vi "fp display engine.vi"(7 "channel data in":sgl[][][](array[numeric]), 10 "Image Refs In":T1[](array[typedef]), 11 "DisplayRefsIn(generic class)":refnum<vi>[](array[refnum])) -> ()   [LabVIEW 2012]
uses:
  <vilib>/vision/Image Controls.llb/IMAQ Image.ctl
  Custom Controls/MAIN Image panel tab Control type def.ctl
  Custom Controls/Ch selector.ctl
  GFG/GFGfpRefGet.vi
  GFG/GFGbooleanGet.vi
  <vilib>/vision/NI_Vision_Development_Module.lvlib
  GFG/GFG library.lvlib
panel:
  in  "ROI colors":u32[](array[colorbox])=[6618880, 16716362, 16860, 16776793, 16750848, 16448250, 16716530, 9567230, 16764108, 7340212, 32639, 0, 13816530, 8421376, 8421631, 7171459, 6618880, 16716362, 16860, 16776793, 16750848, 16448250, 16716530, 9567230, 16764108, 7340212, 32639, 0, 13816530, 8421376, 8421631, 7171459, 6618880, 16716362, 16860, 16776793, 16750848, 16448250, 16716530, 9567230, 16764108, 7340212, 32639, 0, 13816530, 8421376, 8421631, 7171459, 6618880, 16716362, 16860, 16776793, 16750848, 16448250, 16716530, 9567230, 16764108, 7340212, 32639, 0, 13816530, 8421376, 8421631, 7171459, 6618880, 16716362, 16860, 16776793, 16750848, 16448250, 16716530, 9567230, 16764108, 7340212, 32639, 0, 13816530, 8421376, 8421631, 7171459, 6618880, 16716362, 16860, 16776793, 16750848, 16448250, 16716530, 9567230, 16764108, 7340212, 32639, 0, 13816530, 8421376, 8421631, 7171459, 6618880, 16716362, 16860, 16776793, 16750848, 16448250, 16716530, 9567230, 16764108, 7340212, 32639, 0, 13816530, 8421376, 8421631, 7171459, 6618880, 16716362, 16860, 16776793, 16750848, 16448250, 16716530, 9567230, 16764108, 7340212, 32639, 0, 13816530, 8421376, 8421631, 7171459, 6618880, 16716362, 16860, 16776793, 16750848, 16448250, 16716530, 9567230, 16764108, 7340212, 32639, 0, 13816530, 8421376, 8421631, 7171459, 6618880, 16716362, 16860, 16776793, 16750848, 16448250, 16716530, 9567230, 16764108, 7340212, 32639, 0, 13816530, 8421376, 8421631, 7171459, 6618880, 16716362, 16860, 16776793, 16750848, 16448250, 16716530, 9567230, 16764108, 7340212, 32639, 0, 13816530, 8421376, 8421631, 7171459, 6618880, 16716362, 16860, 16776793, 16750848, 16448250, 16716530, 9567230, 16764108, 7340212, 32639, 0, 13816530, 8421376, 8421631, 7171459, 6618880, 16716362, 16860, 16776793, 16750848, 16448250, 16716530, 9567230, 16764108, 7340212, 32639, 0, 13816530, 8421376, 8421631, 7171459, 6618880, 16716362, 16860, 16776793, 16750848, 16448250, 16716530, 9567230, 16764108, 7340212, 32639, 0, 13816530, 8421376, 8421631, 7171459, 6618880, 16716362, 16860, 16776793, 16750848, 16448250, 16716530, 9567230, 16764108, 7340212, 32639, 0, 13816530, 8421376, 8421631, 7171459, 6618880, 16716362, 16860, 16776793, 16750848, 16448250, 16716530, 9567230, 16764108, 7340212, 32639, 0, 13816530, 8421376, 8421631, 7171459, 6618880, 16716362, 16860, 16776793, 16750848, 16448250, 16716530, 9567230, 16764108, 7340212, 32639, 0, 13816530, 8421376, 8421631, 7171459, 6618880, 16716362, 16860, 16776793, 16750848, 16448250, 16716530, 9567230, 16764108, 7340212, 32639, 0, 13816530, 8421376, 8421631, 7171459, 6618880, 16716362, 16860, 16776793, 16750848, 16448250, 16716530, 9567230, 16764108, 7340212, 32639, 0, 13816530, 8421376, 8421631, 7171459, 6618880, 16716362, 16860, 16776793, 16750848, 16448250, 16716530, 9567230, 16764108, 7340212, 32639, 0, 13816530, 8421376, 8421631, 7171459, 6618880, 16716362, 16860, 16776793, 16750848, 16448250, 16716530, 9567230, 16764108, 7340212, 32639, 0, 13816530, 8421376, 8421631, 7171459, 6618880, 16716362, 16860, 16776793, 16750848, 16448250, 16716530, 9567230, 16764108, 7340212, 32639, 0, 13816530, 8421376, 8421631, 7171459, 6618880, 16716362, 16860, 16776793, 16750848, 16448250, 16716530, 9567230, 16764108, 7340212, 32639, 0, 13816530, 8421376, 8421631, 7171459, 6618880, 16716362, 16860, 16776793, 16750848, 16448250, 16716530, 9567230, 16764108, 7340212, 32639, 0, 13816530, 8421376, 8421631, 7171459, 6618880, 16716362, 16860, 16776793, 16750848, 16448250, 16716530, 9567230, 16764108, 7340212, 32639, 0, 13816530, 8421376, 8421631, 7171459]
  out "error out":errorcluster
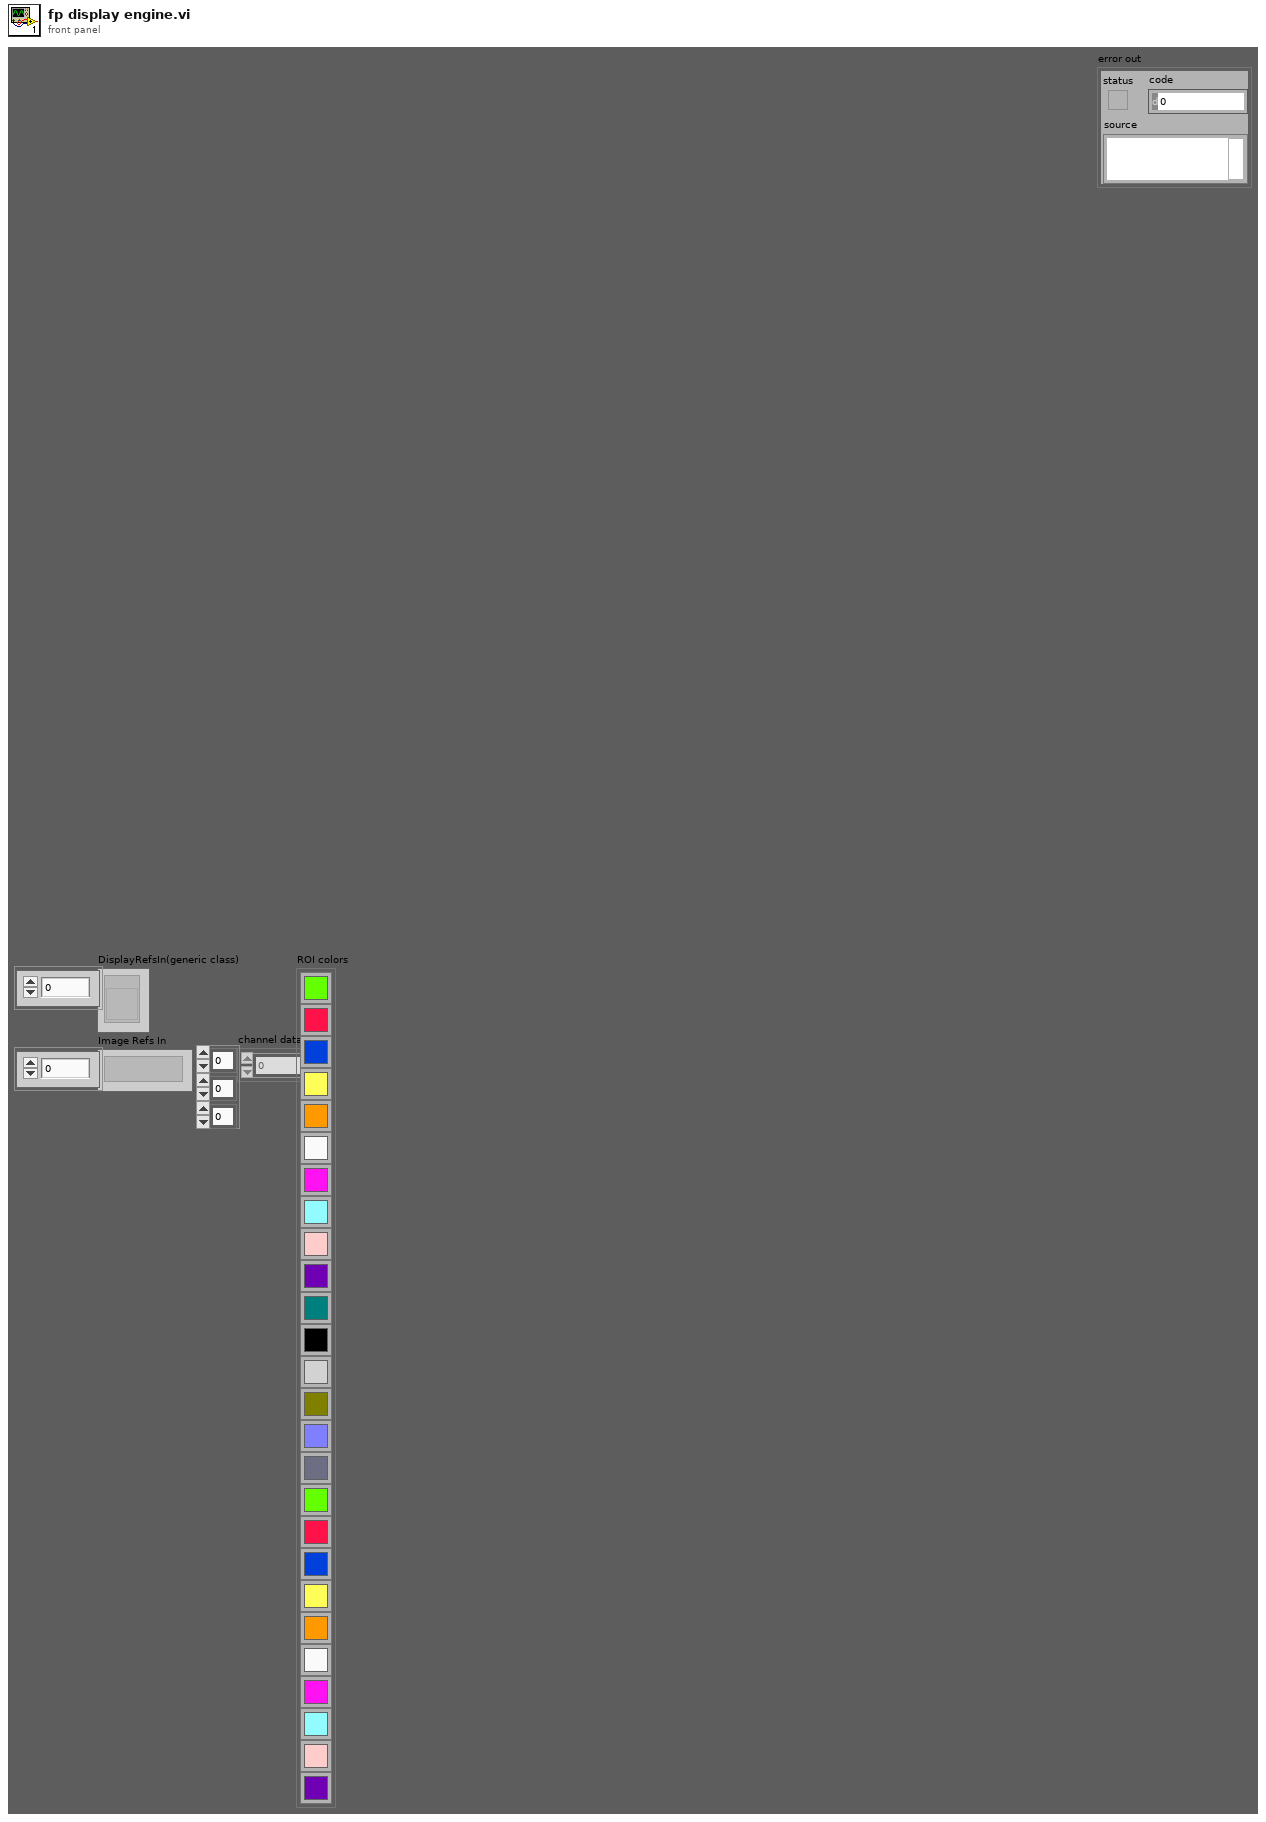
[diagram p1: front panel]
types:
  T1 = typedef "IMAQ Image.ctl" = refnum<image>
  T2 = typedef "MAIN Image panel tab Control type def.ctl" = enum32{"Channel 1", "Channel 2", "Channel 3", "Channel 4", "all channels", "RGB overlay", "ROI", "arbitrary line scan"}
  T3 = enum32{"Channel 1", "Channel 2", "Channel 3", "Channel 4", "Channel 5", "all channels", "RGB overlay", "ROI", "arbitrary line scan"}
  T4 = typedef "Ch selector.ctl" = enum16{"none", "Ch 1", "Ch 2", "Ch 3", "Ch 4", "Ch 5"}
  T5 = typedef "Image Type" = u32
  T6 = cluster{"Global Rectangle":i32[], "Contours":cluster{"Contour Type":u32, "ROI Type":u32, "Points":i32[]}[]}
  T7 = typedef "ROI Descriptor" = cluster{"Global Rectangle":i32[], "Contours":cluster{"ID":enum32{"External", "Internal"}, "Type":u32, "Coordinates":i32[]}[]}
  T8 = cluster{"WaveformChartRef":refnum<vi>, "DigitalRef":refnum<vi>, "ArrayRef":refnum<vi>, "TabControlRef":refnum<vi>, "EnumRef":refnum<vi>, "RingRef":refnum<vi>, "BooleanRef":refnum<vi>, "KnobRef":refnum<vi>, "SlideRef":refnum<vi>, "PathRef":refnum<vi>, "StringRef":refnum<vi>, "ComboBox":refnum<vi>, "WaveformGraphRef":refnum<vi>}
  T9 = cluster{"Mean Value":sgl, "Standard Variation":sgl, "Minimal Value":sgl, "Maximal Value":sgl, "Area (calibrated)":sgl, "Area (pixels)":i32, "%":sgl}[]
  T10 = cluster{"Mean Value":sgl, "Standard Variation":sgl, "Minimal Value":sgl, "Maximal Value":sgl, "Area (calibrated)":sgl, "Area (pixels)":i32, "%":sgl}
  T11 = cluster{"Contour Type":u32, "ROI Type":u32, "Points":i32[]}[]
  T12 = cluster{"Starting Value":sgl, "Incremental Value":sgl, "Histogram":u32[]}
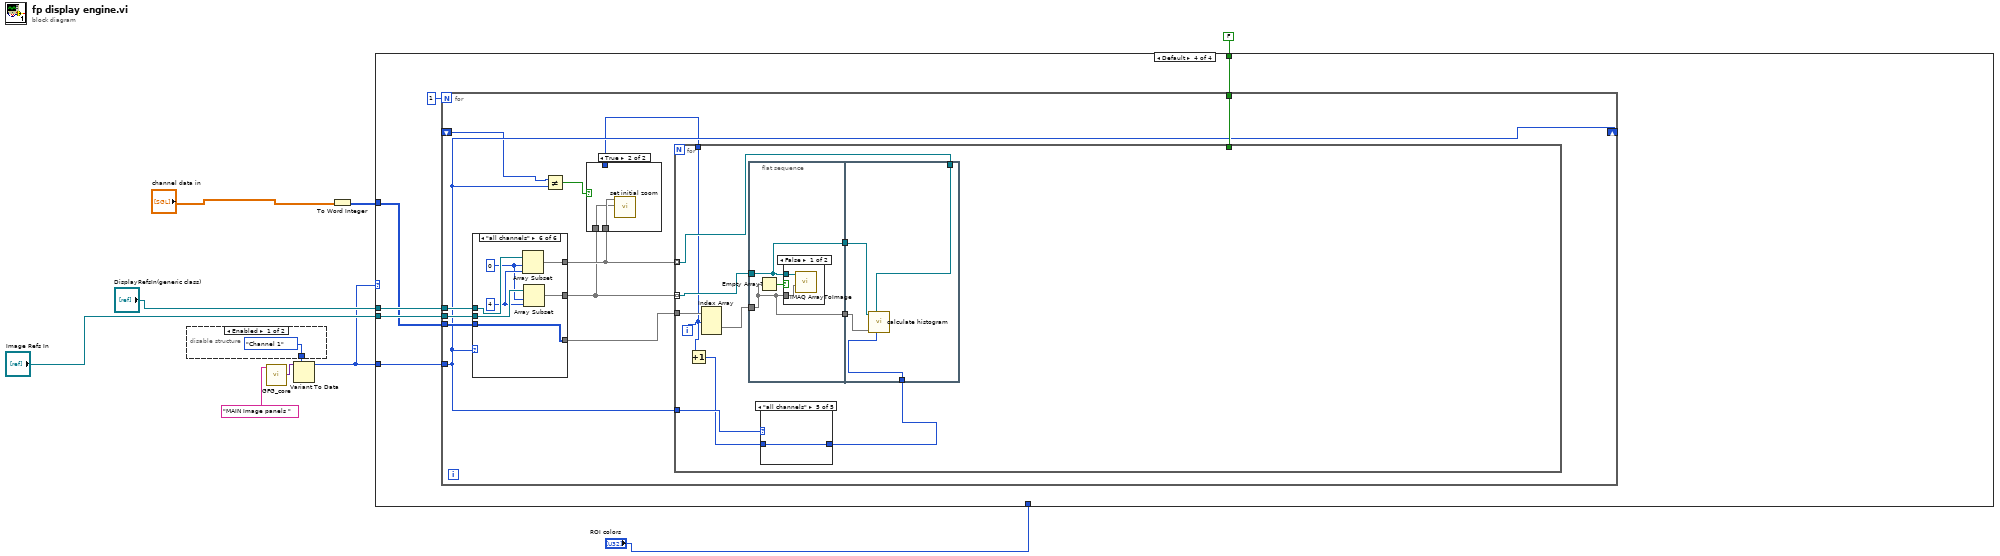
[diagram p0: block diagram]
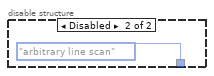
[diagram p2: hidden frame]
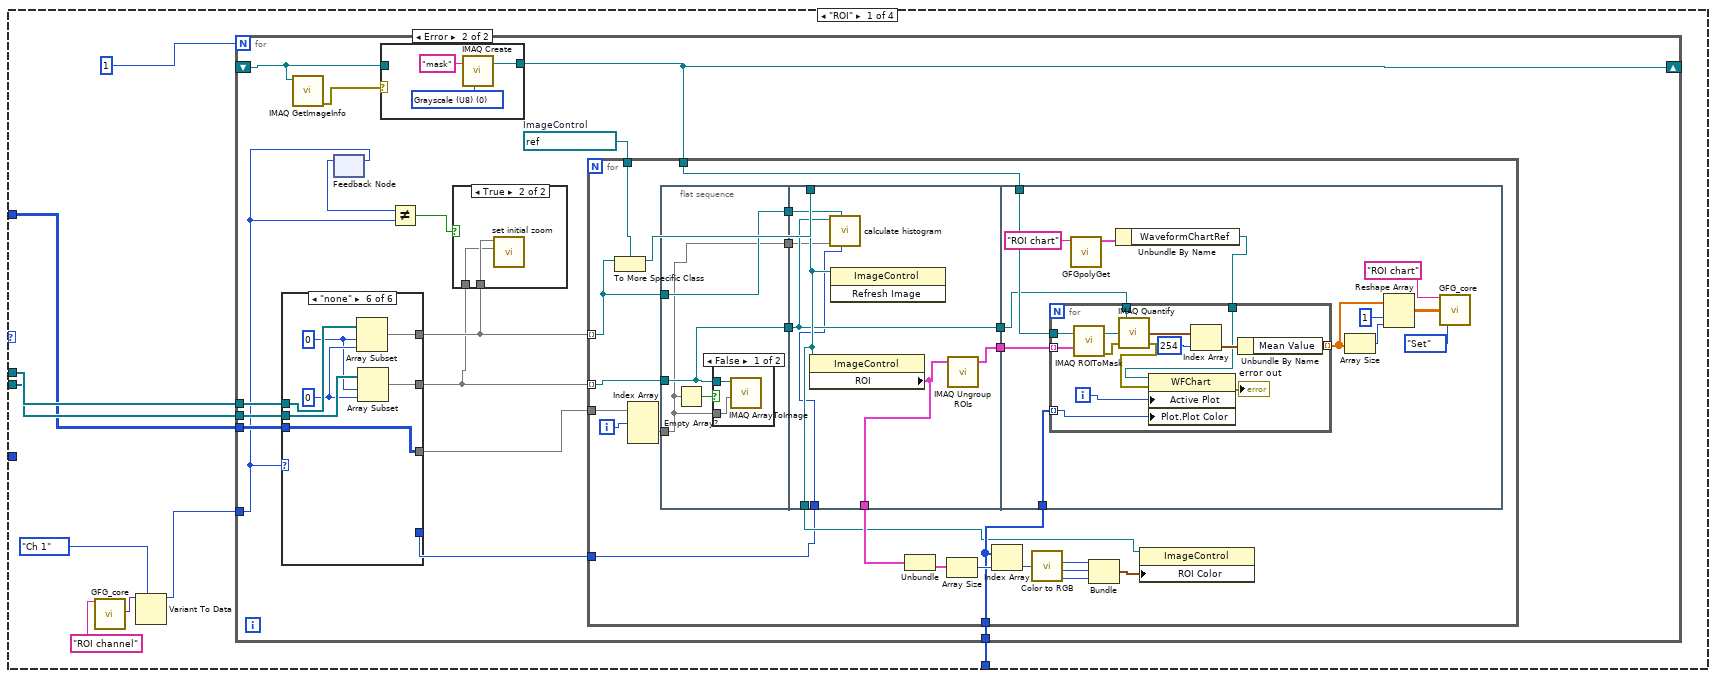
[diagram p3: hidden frame]
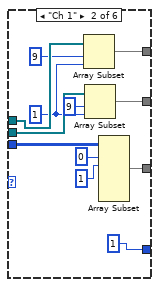
[diagram p7: hidden frame]
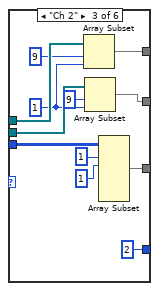
[diagram p8: hidden frame]
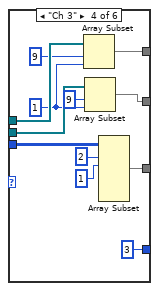
[diagram p9: hidden frame]
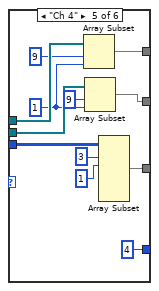
[diagram p10: hidden frame]
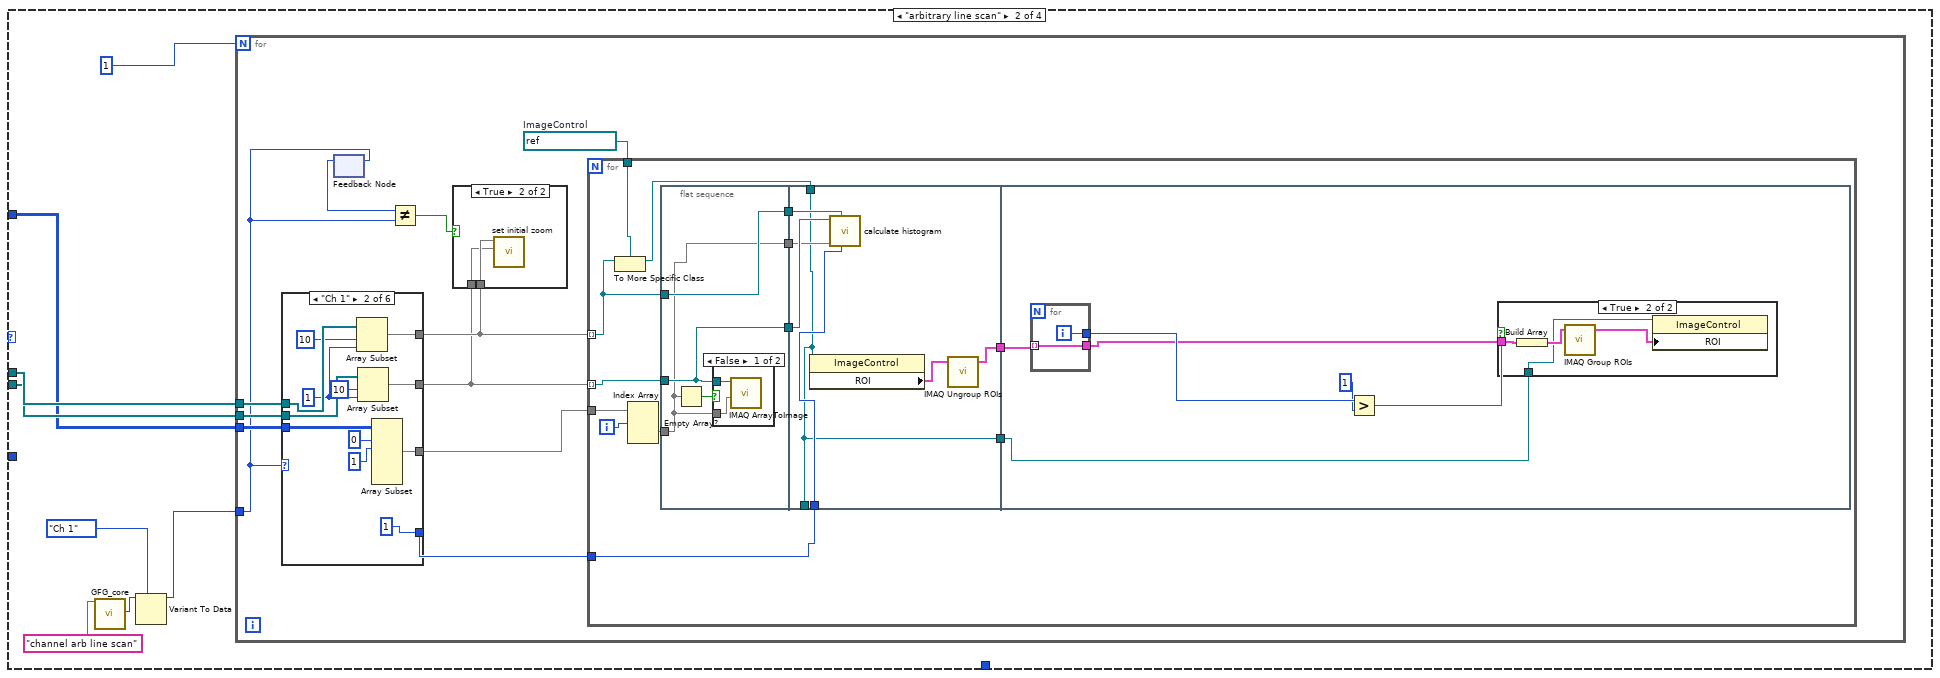
[diagram p12: hidden frame]
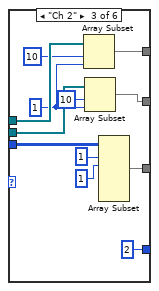
[diagram p15: hidden frame]
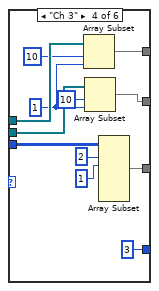
[diagram p16: hidden frame]
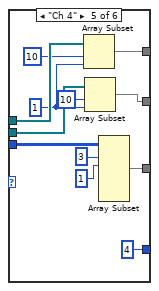
[diagram p17: hidden frame]
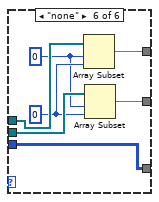
[diagram p18: hidden frame]
diagram:
  n1 = disable-structure shown="Enabled" {
    disable-tunnel: [MAIN_Image_panel_tab_Control_type_def."Channel 1" ("MAIN Image panels") T3."arbitrary line scan" ("MAIN Image panels")] -> w8
    frame Enabled {
    }
    frame Disabled {
    }
  }
  n2 = call "GFG_core.vi"("Variable Name in"="MAIN Image panels ") -> ("Variant Out"=w10:variant)  [unwired: 12 in, 6 out]
  n3 = Variant To Data(type=w8, Variant=w10) -> (data=w4:T2)  [unwired: 1 in, 1 out]
  n4 = To Word Integer(number="channel data in") -> (16bit integer=w3:i16[][][])
  n5 = case shown="Default" w4 {
    tunnel: w4 -> [_ _ _ w356]
    tunnel: "DisplayRefsIn(generic class)" -> [w20 w168 w290 w359]
    tunnel: "Image Refs In" -> [w19 w167 w281 w358]
    tunnel: w3 -> [w18 w166 w289 w357]
    tunnel: FALSE -> [_ _ w288 w354]
    tunnel: "ROI colors" -> [w14 _ _ _]
    frame "ROI" {
      n6 = call "GFG_core.vi"("Variable Name in"="ROI channel") -> ("Variant Out"=w16:variant)  [unwired: 12 in, 6 out]
      n7 = Variant To Data(type=Ch_selector."Ch 1" ("ROI channel"), Variant=w16) -> (data=w15:T4)  [unwired: 1 in, 1 out]
      n8 = for {
        N: 1 -> [_]
        tunnel: w20 -> [w35]
        tunnel: w19 -> [w34]
        tunnel: w18 -> [w33]
        tunnel: w15 -> [w30]
        shift-right: [w27] -> _
        shift-left: _ -> [w26]
        tunnel: w14 -> [w24]
        w32 = refnum<vi> refnum  # ImageControl
        n9 = case shown="\"none\"" w30 {
          tunnel: w35 -> [_ w53 w65 w77 w89 w96]
          tunnel: w34 -> [_ w54 w66 w78 w90 w97]
          tunnel: [_ w50 w62 w74 w86 w93] -> w22
          tunnel: [_ w49 w61 w73 w85 w92] -> w29
          tunnel: w33 -> [_ w48 w58 w70 w82 w91]
          tunnel: [_ w45 w57 w69 w81 w91] -> w36
          tunnel: [_ 1 ("length") 2 ("length") 3 ("length") 4 ("length") _] -> w23
          frame Default {
          }
          frame "Ch 1" {
            w52 = 1 ("length")
            n10 = Array Subset(array=w53, index=9, length=w52) -> (w49:refnum<vi>[])
            n11 = Array Subset(array=w54, index=9, length=w52) -> (w50:T1[])
            n12 = Array Subset(array=w48, index (dim 0)=0 ("index"), length (dim 0)=1 ("length")) -> (w45:i16[][][])  [unwired: 4 in]
          }
          frame "Ch 2" {
            w64 = 1 ("length")
            n13 = Array Subset(array=w65, index=9, length=w64) -> (w61:refnum<vi>[])
            n14 = Array Subset(array=w66, index=9, length=w64) -> (w62:T1[])
            n15 = Array Subset(array=w58, index (dim 0)=1 ("index"), length (dim 0)=1 ("length")) -> (w57:i16[][][])  [unwired: 4 in]
          }
          frame "Ch 3" {
            w75 = 1 ("index")
            n16 = Array Subset(array=w77, index=9, length=w75) -> (w73:refnum<vi>[])
            n17 = Array Subset(array=w78, index=9, length=w75) -> (w74:T1[])
            n18 = Array Subset(array=w70, index (dim 0)=2 ("index"), length (dim 0)=1 ("length")) -> (w69:i16[][][])  [unwired: 4 in]
          }
          frame "Ch 4" {
            w88 = 1 ("index")
            n19 = Array Subset(array=w89, index=9, length=w88) -> (w85:refnum<vi>[])
            n20 = Array Subset(array=w90, index=9, length=w88) -> (w86:T1[])
            n21 = Array Subset(array=w82, index (dim 0)=3 ("index"), length (dim 0)=1 ("length")) -> (w81:i16[][][])  [unwired: 4 in]
          }
          frame "none" {
            w94 = 0 ("index")
            w95 = 0 ("length")
            n22 = Array Subset(array=w96, index=w94, length=w95) -> (w92:refnum<vi>[])
            n23 = Array Subset(array=w97, index=w94, length=w95) -> (w93:T1[])
          }
        }
        n24 = call "IMAQ GetImageInfo"("Image"=w26) -> ("error out"=w25:errorcluster)  [unwired: 3 in, 7 out]
        n25 = feedback-in #1(w30) -> ()
        n26 = feedback #1() -> (w31:T4)  [unwired: 1 in]
        n27 = case shown="Error" w25 {
          tunnel: [w37 w38] -> w27
          tunnel: w26 -> [w37 _]
          frame No Error {
          }
          frame Error {
            w39 = T5 0 items=["Grayscale (U8)", "Grayscale (I16)", "Grayscale (SGL)", "Complex (CSG)", "RGB (U32)", "HSL (U32)", "RGB (U64)"] ("Image Type")
            n28 = call "IMAQ Create"("Image Name"="mask", "Image Type"=w39) -> ("New Image"=w38:T1)  [unwired: 3 in, 1 out]
          }
        }
        n29 = Not Equal?(x=w31, y=w30) -> (x != y?=w28:bool)
        n30 = case shown="True" w28 {
          tunnel: w29 -> [_ w42]
          tunnel: w22 -> [_ w41]
          frame False {
          }
          frame True {
            n31 = call "set initial zoom.vi"("Image Refs In"=w41, "DisplayRefsIn(generic class)"=w42) -> ()  [unwired: 10 in]
          }
        }
        n32 = for {
          tunnel: w29 -> [w100] mode=indexing
          tunnel: w22 -> [w119] mode=indexing
          tunnel: w36 -> [w121]
          tunnel: w32 -> [w118]
          tunnel: w27 -> [w103]
          tunnel: w24 -> [w106]
          tunnel: w23 -> [w98]
          i -> [w116]
          n33 = To More Specific Class(target class=w118, reference=w100) -> (specific class reference=w117:refnum<vi>)  [unwired: 1 in, 1 out]
          n34 = Index Array(array=w121, index (dim 0)=w116) -> (element=w120:i16[][])  [unwired: 2 in]
          n35 = flat-sequence {
            tunnel: w120 -> [w122]
            tunnel: w119 -> [w124]
            tunnel: [w124] -> w104
            tunnel: [w123] -> w101
            tunnel: w100 -> [w123]
            tunnel: [w122] -> w99
            tunnel: w117 -> [w132]
            tunnel: [w134] -> w109
            tunnel: [w133] -> w107
            tunnel: [w130] -> w105
            tunnel: w104 -> [w130]
            tunnel: [w132] -> w102
            tunnel: w101 -> [w131]
            tunnel: w99 -> [w129]
            tunnel: w98 -> [w128]
            tunnel: w107 -> [w144]
            tunnel: w106 -> [w143]
            tunnel: w105 -> [w135]
            tunnel: w103 -> [w136]
            frame #0 {
              n36 = Empty Array?(array=w122) -> (empty?=w125:bool)
              n37 = case shown="False" w125 {
                tunnel: w124 -> [w127 _]
                tunnel: w122 -> [w126 _]
                frame False {
                  n38 = call "IMAQ ArrayToImage"("Image Pixels (I16)"=w126, "Image"=w127) -> ()  [unwired: 8 in, 2 out]
                }
                frame True {
                }
              }
            }
            frame #1 {
              n39 = property class="ImageControl"(reference=w132) -> ("ROI"=w134:T6)  [unwired: 1 in, 2 out]
              n40 = call "calculate histogram.vi"("channel no."=w128, "Image Ctrl Ref (as generic class)"=w131, "Image Array"=w129, "Image"=w130) -> ()  [unwired: 8 in]
              n41 = invoke class="ImageControl" method="Refresh Image"(reference=w132) -> ()  [unwired: 2 in, 3 out]
              n42 = call "IMAQ Ungroup ROIs"("ROI Descriptor"=w134) -> ("ROI Descriptors out"=w133:T7[])  [unwired: 3 in, 1 out]
            }
            frame #2 {
              n43 = call-poly "GFGpolyGet.vi"("Variable Name in"="ROI chart") -> ("output cluster"=w138:T8)  [unwired: 9 in, 1 out]
              n44 = Unbundle By Name(w138) -> ("WaveformChartRef"=w137:refnum<vi>)
              n45 = for {
                tunnel: w135 -> [w161]
                tunnel: w144 -> [w155] mode=indexing
                tunnel: [w157] -> w147 mode=indexing
                tunnel: w136 -> [w154]
                tunnel: w143 -> [w151] mode=indexing
                tunnel: w137 -> [w150]
                i -> [w152]
                n46 = call "IMAQ ROIToMask"("ROI Descriptor"=w155, "Image"=w154) -> ("error out"=w149:errorcluster, "Image Out"=w156:T1)  [unwired: 4 in, 1 out]
                n47 = call "IMAQ Quantify"("error in (no error)"=w149, "Image Mask"=w156, "Image"=w161) -> ("error out"=w148:errorcluster, "Region Reports"=w160:T9)  [unwired: 1 out]
                n48 = property on="Property Node" class="WFChart"(reference=w150, error in=w148, "Active Plot"=w152, "Plot.Plot Color"=w151) -> (error out=→"error out":errorcluster)  [unwired: 1 out]
                n49 = Index Array(array=w160, index=254) -> (element=w158:T10)
                n50 = Unbundle By Name(w158) -> ("Mean Value"=w157:sgl)
              }
              n51 = Array Size(array=w147) -> (size(s)=w146:i32)
              n52 = Reshape Array(w147, 1 ("dimension size"), w146) -> (w141:sgl[][])
              n53 = call "GFG_core.vi"("Variable Name in"="ROI chart", "Variant in"=w141, "Action"=enum16{"Init", "Set", "Get"}."Set") -> ()  [unwired: 10 in, 7 out]
            }
          }
          n54 = Unbundle(w109) -> ("Contours"=w114:T11)  [unwired: 1 out]
          n55 = Array Size(array=w114) -> (size(s)=w115:i32)
          n56 = Index Array(array=w106, index=w115) -> (element=w110:u32)
          n57 = call <vilib>:"Color to RGB.vi"("Color"=w110) -> ("R"=w111:u8, "G"=w112:u8, "B"=w113:u8)  [unwired: 1 out]
          n58 = Bundle("R"=w111, "G"=w112, "B"=w113) -> (w108:cluster{"R":u8, "G":u8, "B":u8})  [unwired: 1 in]
          n59 = property class="ImageControl"(reference=w102, "ROI Color"=w108) -> ()  [unwired: 1 in, 2 out]
        }
      }
    }
    frame "arbitrary line scan" {
      n60 = call "GFG_core.vi"("Variable Name in"="channel arb line scan") -> ("Variant Out"=w164:variant)  [unwired: 12 in, 6 out]
      n61 = Variant To Data(type=Ch_selector."Ch 1" ("ROI channel"), Variant=w164) -> (data=w163:T4)  [unwired: 1 in, 1 out]
      n62 = for {
        N: 1 -> [_]
        tunnel: w168 -> [w179]
        tunnel: w167 -> [w178]
        tunnel: w166 -> [w177]
        tunnel: w163 -> [w174]
        w176 = refnum<vi> refnum  # ImageControl
        n63 = case shown="\"Ch 1\"" w174 {
          tunnel: w179 -> [_ w193 w205 w217 w229 w236]
          tunnel: w178 -> [_ w194 w206 w218 w230 w237]
          tunnel: [_ w190 w202 w214 w226 w233] -> w170
          tunnel: [_ w189 w201 w213 w225 w232] -> w173
          tunnel: w177 -> [_ w188 w198 w210 w222 w231]
          tunnel: [_ w185 w197 w209 w221 w231] -> w180
          tunnel: [_ 1 ("length") 2 ("length") 3 ("length") 4 ("length") _] -> w171
          frame Default {
          }
          frame "Ch 1" {
            w192 = 1 ("length")
            n64 = Array Subset(array=w193, index=10, length=w192) -> (w189:refnum<vi>[])
            n65 = Array Subset(array=w194, index=10, length=w192) -> (w190:T1[])
            n66 = Array Subset(array=w188, index (dim 0)=0 ("index"), length (dim 0)=1 ("length")) -> (w185:i16[][][])  [unwired: 4 in]
          }
          frame "Ch 2" {
            w204 = 1 ("length")
            n67 = Array Subset(array=w205, index=10, length=w204) -> (w201:refnum<vi>[])
            n68 = Array Subset(array=w206, index=10, length=w204) -> (w202:T1[])
            n69 = Array Subset(array=w198, index (dim 0)=1 ("index"), length (dim 0)=1 ("length")) -> (w197:i16[][][])  [unwired: 4 in]
          }
          frame "Ch 3" {
            w215 = 1 ("index")
            n70 = Array Subset(array=w217, index=10, length=w215) -> (w213:refnum<vi>[])
            n71 = Array Subset(array=w218, index=10, length=w215) -> (w214:T1[])
            n72 = Array Subset(array=w210, index (dim 0)=2 ("index"), length (dim 0)=1 ("length")) -> (w209:i16[][][])  [unwired: 4 in]
          }
          frame "Ch 4" {
            w228 = 1 ("index")
            n73 = Array Subset(array=w229, index=10, length=w228) -> (w225:refnum<vi>[])
            n74 = Array Subset(array=w230, index=10, length=w228) -> (w226:T1[])
            n75 = Array Subset(array=w222, index (dim 0)=3 ("index"), length (dim 0)=1 ("length")) -> (w221:i16[][][])  [unwired: 4 in]
          }
          frame "none" {
            w234 = 0 ("index")
            w235 = 0 ("length")
            n76 = Array Subset(array=w236, index=w234, length=w235) -> (w232:refnum<vi>[])
            n77 = Array Subset(array=w237, index=w234, length=w235) -> (w233:T1[])
          }
        }
        n78 = feedback-in #2(w174) -> ()
        n79 = feedback #2() -> (w175:T4)  [unwired: 1 in]
        n80 = Not Equal?(x=w175, y=w174) -> (x != y?=w172:bool)
        n81 = case shown="True" w172 {
          tunnel: w173 -> [_ w182]
          tunnel: w170 -> [_ w181]
          frame False {
          }
          frame True {
            n82 = call "set initial zoom.vi"("Image Refs In"=w181, "DisplayRefsIn(generic class)"=w182) -> ()  [unwired: 10 in]
          }
        }
        n83 = for {
          tunnel: w173 -> [w241] mode=indexing
          tunnel: w170 -> [w248] mode=indexing
          tunnel: w180 -> [w250]
          tunnel: w176 -> [w247]
          tunnel: w171 -> [w239]
          i -> [w245]
          n84 = To More Specific Class(target class=w247, reference=w241) -> (specific class reference=w246:refnum<vi>)  [unwired: 1 in, 1 out]
          n85 = Index Array(array=w250, index (dim 0)=w245) -> (element=w249:i16[][])  [unwired: 2 in]
          n86 = flat-sequence {
            tunnel: w249 -> [w251]
            tunnel: w248 -> [w253]
            tunnel: [w253] -> w243
            tunnel: [w252] -> w242
            tunnel: w241 -> [w252]
            tunnel: [w251] -> w240
            tunnel: w246 -> [w258]
            tunnel: [w263] -> w244
            tunnel: w243 -> [w261]
            tunnel: [w258] -> _
            tunnel: w242 -> [w262]
            tunnel: w240 -> [w260]
            tunnel: w239 -> [w259]
            tunnel: [w258] -> w238
            tunnel: w244 -> [w269]
            tunnel: w238 -> [w268]
            frame #0 {
              n87 = Empty Array?(array=w251) -> (empty?=w254:bool)
              n88 = case shown="False" w254 {
                tunnel: w253 -> [w256 _]
                tunnel: w251 -> [w255 _]
                frame False {
                  n89 = call "IMAQ ArrayToImage"("Image Pixels (I16)"=w255, "Image"=w256) -> ()  [unwired: 8 in, 2 out]
                }
                frame True {
                }
              }
            }
            frame #1 {
              n90 = property class="ImageControl"(reference=w258) -> ("ROI"=w257:T6)  [unwired: 1 in, 2 out]
              n91 = call "calculate histogram.vi"("channel no."=w259, "Image Ctrl Ref (as generic class)"=w262, "Image Array"=w260, "Image"=w261) -> ()  [unwired: 8 in]
              n92 = call "IMAQ Ungroup ROIs"("ROI Descriptor"=w257) -> ("ROI Descriptors out"=w263:T7[])  [unwired: 3 in, 1 out]
            }
            frame #2 {
              n93 = for {
                tunnel: w269 -> [w275] mode=indexing
                tunnel: [w275] -> w264
                tunnel: [w274] -> w267
                i -> [w274]
              }
              n94 = Greater?(x=w267, y=1) -> (0:w265:bool)
              n95 = case shown="True" w265 {
                tunnel: w264 -> [_ w273]
                tunnel: w268 -> [_ w270]
                frame False {
                }
                frame True {
                  n96 = Build Array(w273) -> (w272:T7[])
                  n97 = call "IMAQ Group ROIs"("ROI Descriptors"=w272) -> ("ROI Descriptor out"=w271:T7)  [unwired: 3 in, 1 out]
                  n98 = property class="ImageControl"(reference=w270, "ROI"=w271) -> ()  [unwired: 1 in, 2 out]
                }
              }
            }
          }
        }
      }
    }
    frame "RGB overlay" {
      w276 = refnum<vi> refnum  # ImageControl
      n99 = Array Subset(array=w281, index=8, length=1) -> (w280:T1[])
      n100 = Array Subset(array=w290, index=8, length=1) -> (w277:refnum<vi>[])
      n101 = Array Subset(array=w281, index=0, length=4) -> (w278:T1[])
      n102 = call "set initial zoom.vi"("Image Refs In"=w278, "DisplayRefsIn(generic class)"=w277) -> ()  [unwired: 10 in]
      n103 = for {
        tunnel: w278 -> [w310] mode=indexing
        tunnel: w289 -> [w312]
        tunnel: w288 -> [w303]
        tunnel: [w299] -> w279 mode=indexing
        i -> [w307]
        n104 = Increment(x=w307) -> (x+1=w305:i32)
        n105 = Index Array(array=w312, index (dim 0)=w307) -> (element=w311:i16[][])  [unwired: 2 in]
        n106 = flat-sequence {
          tunnel: w311 -> [w313]
          tunnel: w310 -> [w314]
          tunnel: [w314] -> w308
          tunnel: [w313] -> w306
          tunnel: [w323] -> w309
          tunnel: w308 -> [w323]
          tunnel: w306 -> [w318]
          tunnel: [w321] -> w304
          tunnel: [w318] -> w302
          tunnel: w309 -> [w342]
          tunnel: w305 -> [w341]
          tunnel: w304 -> [w329]
          tunnel: w303 -> [w324]
          tunnel: [w326] -> w300
          tunnel: [w325] -> w301
          frame #0 {
            n107 = Empty Array?(array=w313) -> (empty?=w315:bool)
            n108 = case shown="False" w315 {
              tunnel: w314 -> [w317 _]
              tunnel: w313 -> [w316 _]
              frame False {
                n109 = call "IMAQ ArrayToImage"("Image Pixels (I16)"=w316, "Image"=w317) -> ()  [unwired: 8 in, 2 out]
              }
              frame True {
              }
            }
          }
          frame #1 {
            n110 = Array Max & Min(array=w318) -> (max value=w322:i16, min value=w320:i16)  [unwired: 2 out]
            n111 = Decrement(x=w322) -> (x-1=w319:i16)
            n112 = Bundle(w320, w319) -> (w321:cluster{i16, i16})  [unwired: 1 in]
          }
          frame #2 {
            n113 = Number To Decimal String(number=w341) -> (decimal integer string=w336:string)  [unwired: 1 in]
            n114 = Concatenate Strings("Histogram " ("string"), w336) -> (w344:string)
            n115 = Concatenate Strings("auto scale\n      CH " ("Variable Name in"), w336) -> (w339:string)
            n116 = Concatenate Strings("Min Max Channel " ("Variable Name in"), w336) -> (w327:string)
            n117 = call "IMAQ Histograph"("Image"=w342) -> ("Histogram Graph"=w347:T12)  [unwired: 7 in, 3 out]
            n118 = call-poly "GFGpolyGet.vi"("Variable Name in"=w327) -> ("output cluster"=w338:T8)  [unwired: 9 in, 1 out]
            n119 = call-poly "GFGpolyGet.vi"("Variable Name in"=w339) -> ("Boolean"=w332:bool)  [unwired: 10 in]
            n120 = call-poly "GFGpolyGet.vi"("Variable Name in"=w344) -> ("output cluster"=w345:T8)  [unwired: 9 in, 1 out]
            n121 = Unbundle By Name(w345) -> ("WaveformGraphRef"=w346:refnum<vi>)
            n122 = Unbundle By Name(w338) -> ("SlideRef"=w335:refnum<vi>)
            n123 = property class="WFGraph"(reference=w346, "Value"=w347) -> ()  [unwired: 1 in, 2 out]
            n124 = property class="Slide"(reference=w335) -> (reference out=w330:refnum<vi>, "Value"=w334:variant)  [unwired: 1 in, 1 out]
            n125 = Variant To Data(type=cluster{i32, i32} {0, 2048} ("channel1"), Variant=w334) -> (data=w331:cluster{i32, i32})  [unwired: 1 in, 1 out]
            n126 = Select(t=w329, s=w332, f=w331) -> (s? t:f=w328:cluster{i32, i32})
            n127 = case shown="False" w324 {
              tunnel: w328 -> [w350 w353]
              tunnel: [w349 w351] -> w326
              tunnel: [w348 w352] -> w325
              frame True {
                n128 = Unbundle(w350) -> (w349:i32, w348:i32)
              }
              frame False {
                n129 = Unbundle(w353) -> (w352:i32, w351:i32)
              }
            }
            n130 = property class="Slide"(reference=w330, "Value"=w328) -> ()  [unwired: 1 in, 2 out]
          }
        }
        n131 = Bundle(w302, w301, w300) -> (w299:cluster{i16[][], i32, i32})  [unwired: 1 in]
      }
      n132 = for {
        tunnel: w280 -> [w295] mode=indexing
        tunnel: w279 -> [w294]
        tunnel: w277 -> [w293] mode=indexing
        tunnel: w276 -> [w292]
        n133 = flat-sequence {
          tunnel: w295 -> [w297]
          tunnel: w294 -> [w296]
          tunnel: w291 -> [w298]
          frame #0 {
            n134 = call "overlay3channels.vi"("RGB Overlay"=w297, "Array"=w296) -> ()  [unwired: 10 in]
          }
          frame #1 {
            n135 = invoke class="ImageControl" method="Refresh Image"(reference=w298) -> ()  [unwired: 2 in, 3 out]
          }
        }
        n136 = To More Specific Class(target class=w292, reference=w293) -> (specific class reference=w291:refnum<vi>)  [unwired: 1 in, 1 out]
      }
    }
    frame Default {
      n137 = for {
        N: 1 -> [_]
        tunnel: w359 -> [w369]
        tunnel: w358 -> [w368]
        tunnel: w357 -> [w367]
        tunnel: w356 -> [w362]
        tunnel: w354 -> [w364]
        shift-right: [w362] -> _
        shift-left: _ -> [w361]
        n138 = case shown="\"all channels\"" w362 {
          tunnel: w369 -> [_ w381 w391 w401 w411 w418]
          tunnel: w368 -> [_ w382 w392 w402 w412 w419]
          tunnel: [_ w378 w388 w398 w408 w415] -> w363
          tunnel: [_ w377 w387 w397 w407 w414] -> w366
          tunnel: w367 -> [_ w376 w384 w394 w404 w413]
          tunnel: [_ w373 w383 w393 w403 w413] -> w370
          frame Default {
          }
          frame "Channel 1" {
            w379 = 4 ("index")
            w380 = 1 ("length")
            n139 = Array Subset(array=w381, index=w379, length=w380) -> (w377:refnum<vi>[])
            n140 = Array Subset(array=w382, index=w379, length=w380) -> (w378:T1[])
            n141 = Array Subset(array=w376, index (dim 0)=0 ("index"), length (dim 0)=1 ("length")) -> (w373:i16[][][])  [unwired: 4 in]
          }
          frame "Channel 2" {
            w389 = 5 ("index")
            w390 = 1 ("length")
            n142 = Array Subset(array=w391, index=w389, length=w390) -> (w387:refnum<vi>[])
            n143 = Array Subset(array=w392, index=w389, length=w390) -> (w388:T1[])
            n144 = Array Subset(array=w384, index (dim 0)=1 ("index"), length (dim 0)=1 ("length")) -> (w383:i16[][][])  [unwired: 4 in]
          }
          frame "Channel 3" {
            w399 = 1 ("index")
            w400 = 6 ("index")
            n145 = Array Subset(array=w401, index=w400, length=w399) -> (w397:refnum<vi>[])
            n146 = Array Subset(array=w402, index=w400, length=w399) -> (w398:T1[])
            n147 = Array Subset(array=w394, index (dim 0)=2 ("index"), length (dim 0)=1 ("length")) -> (w393:i16[][][])  [unwired: 4 in]
          }
          frame "Channel 4" {
            w409 = 7 ("index")
            w410 = 1 ("index")
            n148 = Array Subset(array=w411, index=w409, length=w410) -> (w407:refnum<vi>[])
            n149 = Array Subset(array=w412, index=w409, length=w410) -> (w408:T1[])
            n150 = Array Subset(array=w404, index (dim 0)=3 ("index"), length (dim 0)=1 ("length")) -> (w403:i16[][][])  [unwired: 4 in]
          }
          frame "all channels" {
            w416 = 0 ("index")
            w417 = 4 ("length")
            n151 = Array Subset(array=w418, index=w416, length=w417) -> (w414:refnum<vi>[])
            n152 = Array Subset(array=w419, index=w416, length=w417) -> (w415:T1[])
          }
        }
        n153 = Not Equal?(x=w361, y=w362) -> (x != y?=w365:bool)
        n154 = for {
          tunnel: w366 -> [w421] mode=indexing
          tunnel: w363 -> [w424] mode=indexing
          tunnel: w370 -> [w429]
          tunnel: w362 -> [w428]
          tunnel: w364 -> [_]
          tunnel: [w420] -> w360
          i -> [w420]
          n155 = Increment(x=w420) -> (x+1=w427:i32)
          n156 = Index Array(array=w429, index (dim 0)=w420) -> (element=w423:i16[][])  [unwired: 2 in]
          n157 = flat-sequence {
            tunnel: w423 -> [w430]
            tunnel: w424 -> [w431]
            tunnel: [w431] -> w426
            tunnel: [w430] -> w425
            tunnel: w426 -> [w436]
            tunnel: w425 -> [w438]
            tunnel: w422 -> [w437]
            tunnel: w421 -> [w435]
            frame #0 {
              n158 = Empty Array?(array=w430) -> (empty?=w432:bool)
              n159 = case shown="False" w432 {
                tunnel: w431 -> [w434 _]
                tunnel: w430 -> [w433 _]
                frame False {
                  n160 = call "IMAQ ArrayToImage"("Image Pixels (I16)"=w433, "Image"=w434) -> ()  [unwired: 8 in, 2 out]
                }
                frame True {
                }
              }
            }
            frame #1 {
              n161 = call "calculate histogram.vi"("channel no."=w437, "Image Ctrl Ref (as generic class)"=w435, "Image Array"=w438, "Image"=w436) -> ()  [unwired: 8 in]
            }
          }
          n162 = case shown="\"all channels\"" w428 {
            tunnel: [1 2 3 4 w443] -> w422
            tunnel: w427 -> [_ _ _ _ w443]
            frame "Channel 1", Default {
            }
            frame "Channel 2" {
            }
            frame "Channel 3" {
            }
            frame "Channel 4" {
            }
            frame "all channels" {
            }
          }
        }
        n163 = case shown="True" w365 {
          tunnel: w366 -> [_ w372]
          tunnel: w363 -> [_ w371]
          tunnel: w360 -> [_ _]
          frame False {
          }
          frame True {
            n164 = call "set initial zoom.vi"("Image Refs In"=w371, "DisplayRefsIn(generic class)"=w372) -> ()  [unwired: 10 in]
          }
        }
      }
    }
  }
